vi "Init.vi"(8 "Error In":errorcluster, 10 "Folder Path":path, 11 "Plugin Framework In":refnum<class "File Parser Interface.lvclass">) -> (0 "Error Out":errorcluster, 3 "File Parser Interface out":refnum<class "File Parser Interface.lvclass">)   [LabVIEW 2018, in "File Parser Interface.lvlib" / "File Parser Interface.lvclass"]
uses:
  File Parser Interface.lvclass
  FPF.lvlibp/Factory Plugin Framework.lvclass
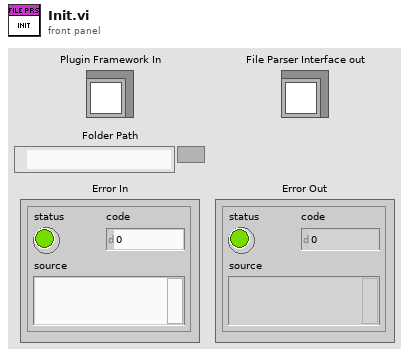
[diagram p1: front panel]
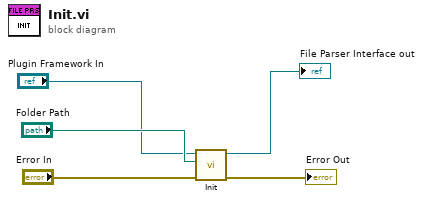
[diagram p0: block diagram]
diagram:
  n1 = call-parent "Init.vi"("Error In"="Error In", "Folder Path"="Folder Path", "Plugin Framework In"="Plugin Framework In") -> ("Error Out"=→"Error Out":errorcluster, "Factory Plugin Framework out"=→"File Parser Interface out":refnum<class "File Parser Interface.lvclass">)  [unwired: 7 in]
